vi "Measure.vi"(8 "error in":errorcluster, 10 "AI duration (ms)":i32=1000, 11 "Resources in":T1={"ZI Handle"={"handleValid"=FALSE, "Conn"=0, "Path Prefix"="", "Handle"=0, "Clockbase(s)"=0.0, "Connected"=FALSE}, "ZI ModHandle"={"handleValid"=FALSE, "Conn"=0, "ModHandle"=0, "moduleID"="", "Path Prefix"=""}, "VISA Keithley"="KEITHLEY"} {"ZI ModHandle"."ModHandle" format="0x%08x"; "ZI ModHandle"."Conn" format="0x%08x"; "ZI Handle"."Handle" format="0x%08x"; "ZI Handle"."Conn" format="0x%08x"}) -> (0 "error out":errorcluster, 1 "data":waveform(dbl), 2 "progress":dbl(slide) scale=0.0..1.0, 3 "Resources out":T1 {"ZI ModHandle"."ModHandle" format="0x%08x"; "ZI ModHandle"."Conn" format="0x%08x"; "ZI Handle"."Handle" format="0x%08x"; "ZI Handle"."Conn" format="0x%08x"})   [LabVIEW 2021]
uses:
  Main/Ver_2/Resources_v2.ctl
  <instrlib>/Zurich Instruments LabOne/Public/ziTypeHandle.ctl
  <instrlib>/Zurich Instruments LabOne/Public/Modules/ziTypeModHandle.ctl
  <vilib>/Utility/error.llb/Error Cluster From Error Code.vi
  <vilib>/ErrorRing/Error Ring.xnode
  <instrlib>/Zurich Instruments LabOne/Zurich Instruments LabOne.lvlib
panel:
  in  "Timeout [ms]":u64=5000 min=4000
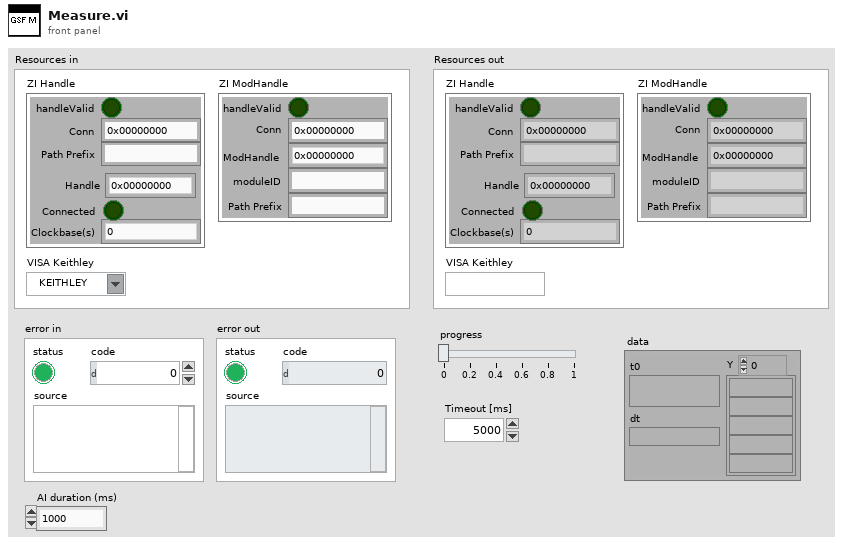
[diagram p1: front panel]
types:
  T1 = typedef "Resources_v2.ctl" = cluster{"ZI Handle":T2, "ZI ModHandle":T3, "VISA Keithley":refnum<visa-resource-name>}
  T2 = typedef "Zurich Instruments LabOne.lvlib/ziTypeHandle.ctl" = cluster{"handleValid":bool, "Conn":u64, "Path Prefix":string, "Handle":u64, "Clockbase(s)":dbl, "Connected":bool}
  T3 = typedef "Zurich Instruments LabOne.lvlib/ziTypeModHandle.ctl" = cluster{"handleValid":bool, "Conn":u64, "ModHandle":u64, "moduleID":string, "Path Prefix":string}
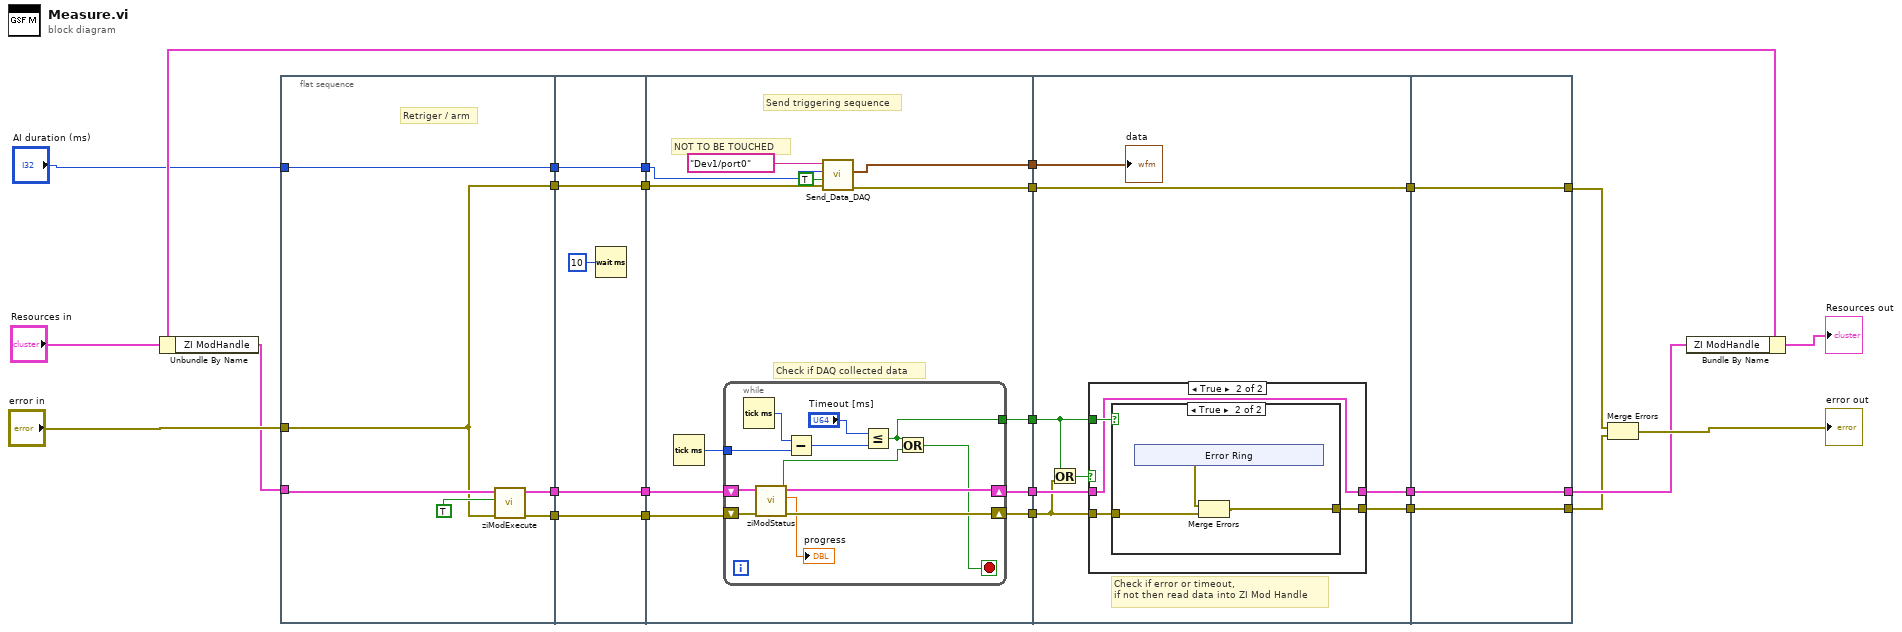
[diagram p0: block diagram]
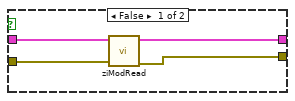
[diagram p2: hidden frame]
diagram:
  n1 = Unbundle By Name("Resources in") -> ("ZI ModHandle"=w5:T3)
  n2 = flat-sequence {
    tunnel: w5 -> [w31]
    tunnel: "error in" -> [w27]
    tunnel: [w27] -> w20
    tunnel: [w29] -> w19
    tunnel: [w28] -> w18
    tunnel: "AI duration (ms)" -> [w26]
    tunnel: [w26] -> w17
    tunnel: [w35] -> w16
    tunnel: w20 -> [w35]
    tunnel: [w34] -> w15
    tunnel: w19 -> [w34]
    tunnel: [w33] -> w14
    tunnel: w18 -> [w33]
    tunnel: [w32] -> w13
    tunnel: w17 -> [w32]
    tunnel: w16 -> [w42]
    tunnel: w15 -> [w48]
    tunnel: w14 -> [w47]
    tunnel: [w41] -> w12
    tunnel: [w45] -> w11
    tunnel: [w44] -> w10
    tunnel: [w43] -> w9
    tunnel: w13 -> [w39]
    tunnel: [w37] -> w1
    tunnel: w12 -> [w68]
    tunnel: w11 -> [w66]
    tunnel: w10 -> [w65]
    tunnel: w9 -> [w62]
    tunnel: [w68] -> w8
    tunnel: [w64] -> w7
    tunnel: [w63] -> w6
    tunnel: w1 -> [w61]
    tunnel: [w87] -> w3
    tunnel: [w88] -> w4
    tunnel: w8 -> [w86]
    tunnel: w7 -> [w88]
    tunnel: w6 -> [w87]
    tunnel: [w86] -> w2
    frame #0 {
      # "Retriger / arm"
      n3 = call <instrlib>:"ziModExecute.vi"("Error In"=w27, "Modal (F)"=TRUE, "ziModHandle In"=w31) -> ("Error Out"=w28:errorcluster, "ziModHandle Out"=w29:T3)  [unwired: 6 in]
    }
    frame #1 {
      n4 = Wait (ms)(milliseconds to wait=u32 10) -> ()  [unwired: 1 out]
    }
    frame #2 {
      # "NOT TO BE TOUCHED"
      # "Check if DAQ collected data"
      # "Send triggering sequence"
      n5 = Tick Count (ms)() -> (millisecond timer value=w46:u32)
      n6 = while {
        shift-right: [w59] -> w44
        shift-left: w48 -> [w60]
        shift-right: [w57] -> w43
        shift-left: w47 -> [w58]
        tunnel: w46 -> [w54]
        tunnel: [w49] -> w45
        stop <- w50 stop-if-true
        n7 = Tick Count (ms)() -> (millisecond timer value=w55:u32)
        n8 = call <instrlib>:"ziModStatus.vi"("Error In"=w58, "ModHandle IN"=w60) -> ("Error Out"=w57:errorcluster, "Finished?"=w51:bool, "Progress (unity)"=→"progress":dbl, "ModHandle Out"=w59:T3)  [unwired: 5 in]
        n9 = Subtract(x=w55, y=w54) -> (x-y=w53:u32)
        n10 = Less Or Equal?(x="Timeout [ms]", y=w53) -> (x <= y?=w49:bool)
        n11 = Or(x=w49, y=w51) -> (x .or. y?=w50:bool)
      }
      n12 = call "Send_Data_DAQ.vi"("error in"=w42, "AI Trig"=TRUE, "AI duration (ms)"=w39, "Digital Ports"=tag "Dev1/port0") -> ("error out"=w41:errorcluster, "data"=w37:waveform(dbl))  [unwired: 6 in]
    }
    frame #3 {
      # "Check if error or timeout,\nif not then read data into ZI Mod Handle"
      n13 = Or(x=w66, y=w62) -> (x .or. y?=w67:bool)
      n14 = case shown="True" w67 {
        tunnel: w62 -> [w71 w75]
        tunnel: w66 -> [_ w76]
        tunnel: [w70 w74] -> w63
        tunnel: w65 -> [w72 w73]
        tunnel: [w69 w73] -> w64
        frame False {
          n15 = call <instrlib>:"ziModRead.vi"("error in"=w71, "ziModHandle In"=w72) -> ("error out"=w70:errorcluster, "ziModHandle Out"=w69:T3)  [unwired: 8 in]
        }
        frame True {
          n16 = case shown="True" w76 {
            tunnel: w75 -> [w77 w79]
            tunnel: [w77 w78] -> w74
            frame False {
            }
            frame True {
              n17 = xnode "Error Ring"() -> ("error out"=w80:errorcluster)
              n18 = Merge Errors(w80, w79) -> (w78:errorcluster)
            }
          }
        }
      }
      "data" <- w61
    }
    frame #4 {
    }
  }
  n19 = Merge Errors(w2, w3) -> (→"error out":errorcluster)
  n20 = Bundle By Name(cluster="Resources in", "ZI ModHandle"=w4) -> (→"Resources out":T1)
